vi "File.Excel, Read Worksheet to 2D Str.vi"(8 "error in (no error)":errorcluster, 10 "Worksheet Index":i32, 11 "Excel File Path":path) -> (0 "error out":errorcluster, 3 "Data":string[][](array[string]))   [LabVIEW 2019]
uses:
  <vilib>/Utility/NIReport.llb/Report Type.ctl
  <vilib>/addons/_office/excel.llb/Excel Get Data ([str]).vi
  <vilib>/Utility/NIReport.llb/NI_report.lvclass
  <vilib>/Utility/NIReport.llb/Excel/NI_Excel.lvclass
  <vilib>/Utility/NIReport.llb/NI_ReportGenerationCore.lvlib
  <vilib>/addons/_office/NI_ReportGenerationToolkit.lvlib
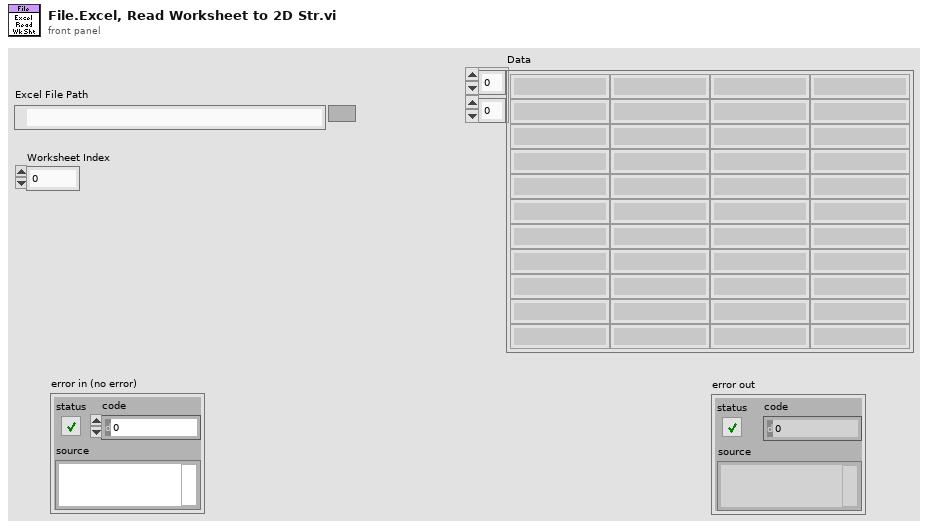
[diagram p1: front panel]
types:
  T1 = typedef "NI_ReportGenerationCore.lvlib/Report Type.ctl" = enum16{"HTML", "Word", "Excel"}
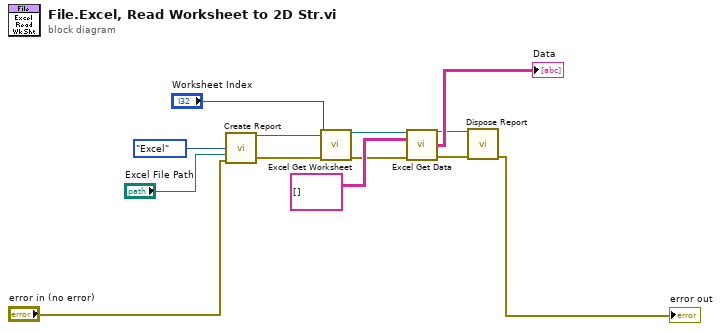
[diagram p0: block diagram]
diagram:
  n1 = call <vilib>:"Create Report.vi"("report type"=Report_Type."Excel", "template (empty)"="Excel File Path", "error in (no error)"="error in (no error)") -> ("report out"=w13:refnum<class "NI_report.lvclass">, "error out"=w10:errorcluster)  [unwired: 11 in]
  n2 = call <vilib>:"Excel Get Worksheet.vi"("report in"=w13, "worksheet index (0)"="Worksheet Index", "error in (no error)"=w10) -> ("report out"=w8:refnum<class "NI_report.lvclass">, "error out"=w3:errorcluster)  [unwired: 11 in]
  n3 = call-poly <vilib>:"Excel Get Data.vi"("report in"=w8, "data type"=string[][] [] ("Data"), "error in (no error)"=w3) -> ("report out"=w5:refnum<class "NI_report.lvclass">, "data"=→"Data":string[][], "error out"=w4:errorcluster)  [unwired: 10 in]
  n4 = call-dynamic "Dispose Report.vi"("report in"=w5, "error in (no error)"=w4) -> ("error out"=→"error out":errorcluster)  [unwired: 13 in]
